vi "Get Class Version from Type Descriptor.vi"(8 "error in":errorcluster, 10 "data string":string, 11 "type string":i16[](array[numeric])) -> (0 "error out":errorcluster, 2 "Version":T1)   [LabVIEW 2020, in "JKI JSON Object Serialization.lvlib" / "OOP_Utility.lvlib" / "Reflection.lvclass"]
uses:
  Reflection.lvclass
  Reflection.lvclass/Reflection.ctl
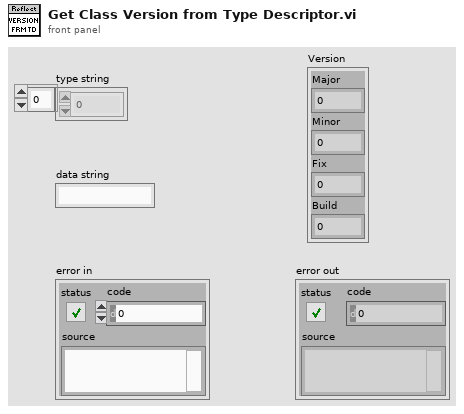
[diagram p1: front panel]
types:
  T1 = cluster{"Major":u16, "Minor":u16, "Fix":u16, "Build":u16}
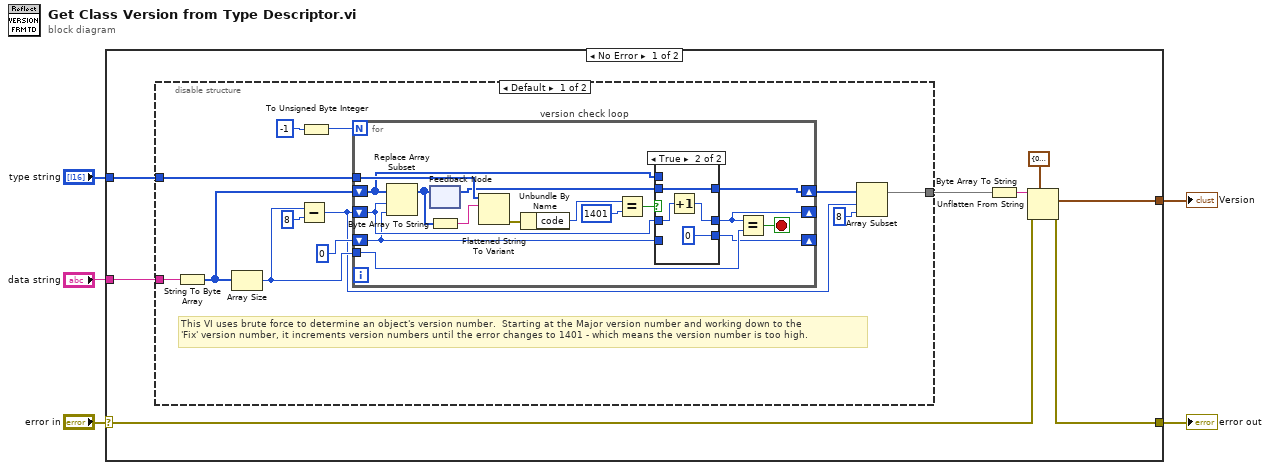
[diagram p0: block diagram]
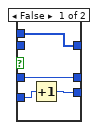
[diagram p2: hidden frame]
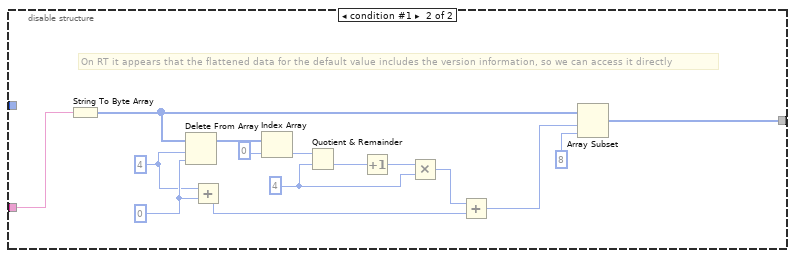
[diagram p3: hidden frame]
diagram:
  n1 = case shown="No Error" "error in" {
    selector: "error in" -> [w7 w65]
    tunnel: "data string" -> [w13 _]
    tunnel: "type string" -> [w12 _]
    tunnel: [w8 _] -> w3
    tunnel: [w6 w65] -> w5
    frame No Error {
      n2 = disable-structure shown="Default" {
        disable-tunnel: w13 -> [w24 w50]
        disable-tunnel: w12 -> [w22 _]
        disable-tunnel: [w14 w51] -> w11
        frame condition #0 (active) {
          # "This VI uses brute force to determine an object's version number.  Starting at the Major version number and working down to the\n'Fix' version number, it increments version numbers until the error changes to 1401 - which means the version number is too high."
          n3 = String To Byte Array(string=w24) -> (unsigned byte array=w23:u8[])
          n4 = Array Size(array=w23) -> (size(s)=w19:i32)
          n5 = Subtract(x=w19, y=8) -> (x-y=w16:i32)
          n6 = To Unsigned Byte Integer(number=i8 -1) -> (unsigned 8bit integer=w20:u8)
          n7 = for "version check loop" {
            N: w20 -> [_]
            tunnel: w22 -> [w40]
            shift-right: [w32] -> w17
            shift-left: w23 -> [w36]
            shift-right: [w30] -> _
            shift-left: w16 -> [w31]
            tunnel: w19 -> [w29]
            shift-right: [w26] -> _
            shift-left: u8 0 ("unsigned 8bit integer") -> [w27]
            stop <- w28 stop-if-true
            n8 = Replace Array Subset(array=w36, new element=w27, index=w31) -> (w35:u8[])
            n9 = feedback #1() -> (w34:u8[])  [unwired: 1 in]
            n10 = feedback-in #1(w35) -> ()
            n11 = Byte Array To String(unsigned byte array=w35) -> (string=w41:string)
            n12 = Flattened String To Variant(6:w41, 7:w40) -> (0:w37:errorcluster)  [unwired: 1 in, 1 out]
            n13 = Unbundle By Name(w37) -> ("code"=w39:i32)
            n14 = Equal?(x=w39, y=1401) -> (x = y?=w33:bool)
            n15 = case shown="True" w33 {
              tunnel: w36 -> [w45 _]
              tunnel: w34 -> [_ w49]
              tunnel: [w45 w49] -> w32
              tunnel: w31 -> [w44 w48]
              tunnel: [w44 w47] -> w30
              tunnel: w27 -> [w43 _]
              tunnel: [w42 u8 0 ("unsigned 8bit integer")] -> w26
              frame False {
                n16 = Increment(x=w43) -> (x+1=w42:u8)
              }
              frame True {
                n17 = Increment(x=w48) -> (x+1=w47:i32)
              }
            }
            n18 = Equal?(x=w30, y=w29) -> (x = y?=w28:bool)
          }
          n19 = Array Subset(array=w17, index=w16, length=8) -> (w14:u8[])
        }
        frame condition #1 {
          w59 = u8 4 ("y")
          w53 = 0 ("index")
          w52 = 4 ("offset (0)")
          # "On RT it appears that the flattened data for the default value includes the version information, so we can access it directly"
          n20 = String To Byte Array(string=w50) -> (unsigned byte array=w55:u8[])
          n21 = Delete From Array(array=w55, length=w52, index=w53) -> (array with subset deleted=w57:u8[])  [unwired: 1 out]
          n22 = Add(x=w52, y=w53) -> (x+y=w54:i32)
          n23 = Index Array(array=w57, index=0) -> (element=w62:u8)
          n24 = Quotient & Remainder(x=w62, y=w59) -> (floor(x/y)=w61:u8)  [unwired: 1 out]
          n25 = Increment(x=w61) -> (x+1=w60:u8)
          n26 = Multiply(x=w60, y=w59) -> (x*y=w58:u8)
          n27 = Add(x=w58, y=w54) -> (x+y=w56:i32)
          n28 = Array Subset(array=w55, index=w56, length=8) -> (w51:u8[])
        }
      }
      n29 = Byte Array To String(unsigned byte array=w11) -> (string=w10:string)
      n30 = Unflatten From String(type=T1 {"Major"=0, "Minor"=0, "Fix"=0, "Build"=0} ("Version"), binary string=w10, error in (no error)=w7) -> (value=w8:T1, error out=w6:errorcluster)  [unwired: 2 in, 1 out]
    }
    frame Error {
    }
  }
  "error out" <- w5
  "Version" <- w3
